vi "Stop Core.vi"(10 "final error code":i32, 11 "Camera in":refnum<class "Camera.lvclass">) -> (3 "Camera out":refnum<class "Camera.lvclass">)   [LabVIEW 2021, in "Camera.lvlib" / "Camera.lvclass"]
doc: "(<B>Filename</B>: Actor Framework.lvlib:Actor.lvclass:Stop Core.vi)\n\nDefines what the actor does before it stops. Use the <B>final error code</B> input to determine whether the actor shut down in response to an error.\n\nBy default, this method does nothing. A descendant class may override it to define behavior, such as shutting down any processes the actor initiated in its override of the Actor Core method."
uses:
  Camera.lvclass
  Camera.lvclass/Camera.ctl
  Utilities/RWC_Actions.ctl
  <vilib>/ActorFramework/Actor/Actor.lvclass
panel:
  out "Cam inner parameters":T1
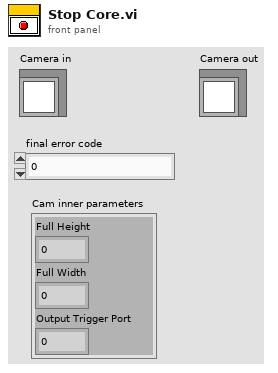
[diagram p1: front panel]
types:
  T1 = cluster{"Full Height":dbl, "Full Width":dbl, "Output Trigger Port":dbl}
  T2 = typedef "RWC_Actions.ctl" = enum16{"Read", "Write", "Read and Create"}
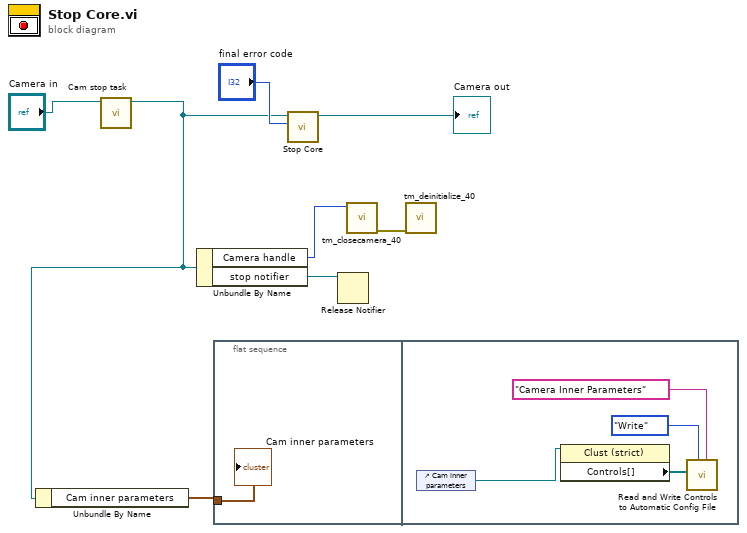
[diagram p0: block diagram]
diagram:
  n1 = call "Cam stop task.vi"("Camera in"="Camera in") -> ("Camera out"=w1:refnum<class "Camera.lvclass">)  [unwired: 9 in, 1 out]
  n2 = Unbundle By Name(w1) -> ("Cam inner parameters"=w3:T1)
  n3 = Unbundle By Name(w1) -> ("Camera handle"=w5:u32, "stop notifier"=w6:refnum<notifier>)
  n4 = flat-sequence {
    tunnel: w3 -> [w9]
    frame #0 {
      "Cam inner parameters" <- w9
    }
    frame #1 {
      n5 = control-ref of="Cam inner parameters"() -> (w10:refnum<vi>)
      n6 = property class="Clust (strict)"(reference=w10) -> ("Controls[]"=w11:refnum<vi>[])  [unwired: 1 in, 2 out]
      n7 = call "Read and Write Controls to Automatic Config File.vi"("file name"="Camera Inner Parameters" ("section (optional)"), "Action"=RWC_Actions."Write", "Control References"=w11) -> ()  [unwired: 8 in, 1 out]
    }
  }
  n8 = call-parent "Stop Core.vi"("final error code"="final error code", "Actor in"=w1) -> ("Actor out"=→"Camera out":refnum<class "Camera.lvclass">)  [unwired: 9 in]
  n9 = Release Notifier(notifier=w6) -> ()  [unwired: 2 in, 3 out]
  n10 = call <userlib>:"tm_closecamera_40.vi"("Handle in"=w5) -> ("error out"=w4:errorcluster)  [unwired: 10 in]
  n11 = call <userlib>:"tm_deinitialize_40.vi"("error in (no error)"=w4) -> ()  [unwired: 10 in, 1 out]
